vi "move curve.vi"(8 "错误输入（无错误）":errorcluster, 9 "XY":cluster{"X":dbl, "Y":dbl}, 11 "引用":refnum<vi>) -> (0 "错误输出":errorcluster, 3 "引用输出":refnum<vi>)   [LabVIEW 2011]
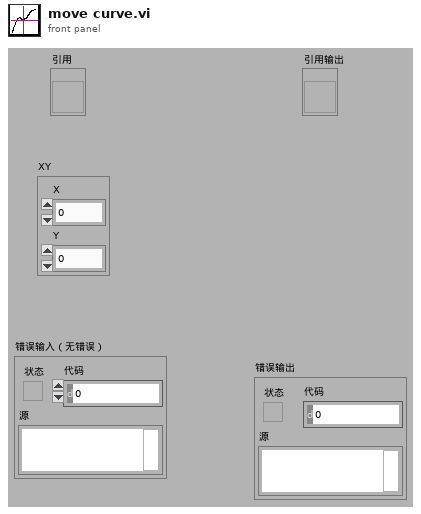
[diagram p1: front panel]
types:
  T1 = cluster{"Font Name:":string, "Size":i16, "Strikeout?":bool, "Italic?":bool, "Underline?":bool, "Outline?":bool, "Shadow?":bool, "Bold?":bool}
  T2 = typedef "LVPoint32TypeDef.ctl" = cluster{"Horizontal":i32, "Vertical":i32}
  T3 = typedef "LVRectTypeDef.ctl" = cluster{"left":i16, "top":i16, "right":i16, "bottom":i16}
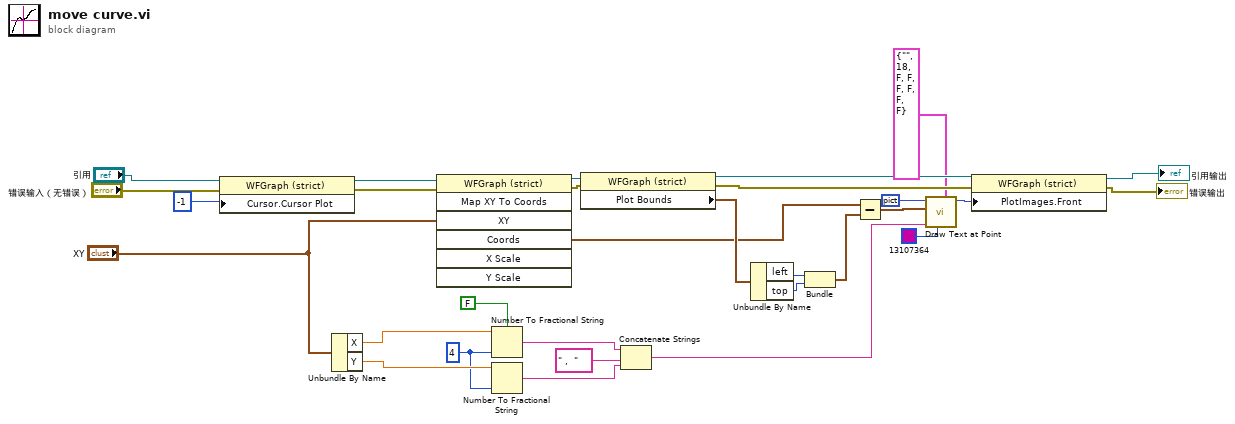
[diagram p0: block diagram]
diagram:
  w8 = i16 4 ("宽度(-)")
  n1 = property class="WFGraph (strict)"(reference="引用", error in="错误输入（无错误）", "Cursor.Cursor Plot"=-1 ("游标.游标关联曲线")) -> (reference out=w25:refnum<vi>, error out=w19:errorcluster)
  n2 = Unbundle By Name("XY") -> ("X"=w16:dbl, "Y"=w15:dbl)
  n3 = invoke class="WFGraph (strict)" method="Map XY To Coords"(reference=w25, error in=w19, "XY"="XY") -> (reference out=w24:refnum<vi>, error out=w18:errorcluster, "Coords"=w23:T2)  [unwired: 4 in, 4 out]
  n4 = Number To Fractional String(use system decimal point (T)=FALSE ("使用系统小数点(T)"), number=w16, precision (6)=w8) -> (F-format string=w14:string)  [unwired: 1 out]
  n5 = Number To Fractional String(number=w15, precision (6)=w8) -> (F-format string=w12:string)  [unwired: 2 out]
  n6 = property class="WFGraph (strict)"(reference=w24, error in=w18) -> (reference out=w21:refnum<vi>, error out=w20:errorcluster, "Plot Bounds"=w29:T3)
  n7 = Concatenate Strings(w14, " ,  " ("字符串"), w12) -> (w11:string)
  n8 = Unbundle By Name(w29) -> ("left"=w28:i16, "top"=w27:i16)
  n9 = Bundle("left"=w28, "top"=w27) -> (w26:cluster{"left":i16, "top":i16})  [unwired: 1 out]
  n10 = Subtract(x=w23, y=w26) -> (x-y=w10:T2)
  n11 = call <vilib>:"Draw Text at Point.vi"("[user-specified font]"=T1 {"Font Name:"="", "Size"=18, "Strikeout?"=FALSE, "Italic?"=FALSE, "Underline?"=FALSE, "Outline?"=FALSE, "Shadow?"=FALSE, "Bold?"=FALSE}, "text color(black)"=u32 13107364, "text"=w11, "origin"=w10, "picture"=picture data[5B]) -> ("new picture"=w17:picture)  [unwired: 4 in, 2 out]
  n12 = property class="WFGraph (strict)"(reference=w21, error in=w20, "PlotImages.Front"=w17) -> (reference out=→"引用输出":refnum<vi>, error out=→"错误输出":errorcluster)
